vi "_lvcicd_dependencies-Post-Install Custom Action.vi"(10 "Variant":variant) -> (0 "error out":errorcluster)   [LabVIEW 2014]
panel:
  out "data":T1(ring)
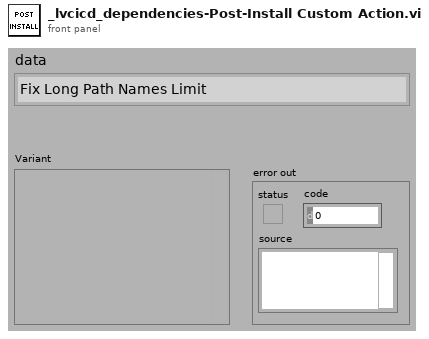
[diagram p1: front panel]
types:
  T1 = enum16{"Fix Long Path Names Limit", "Fix Running Scripts Is Disabled", "-- Exit ---"}
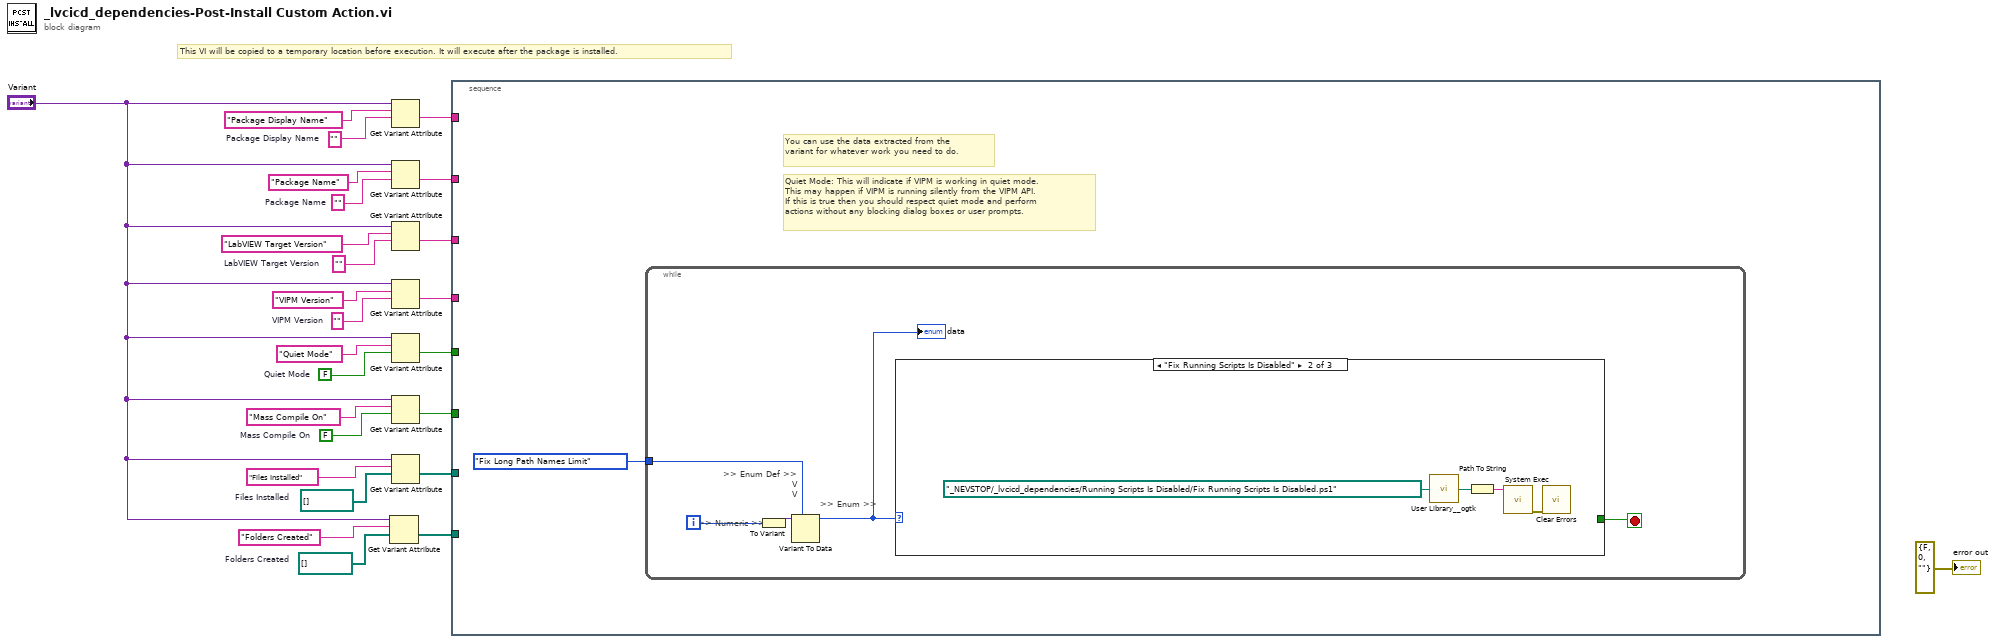
[diagram p0: block diagram]
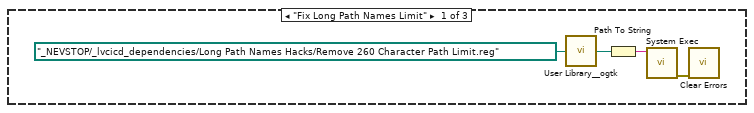
[diagram p2: hidden frame]
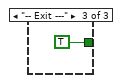
[diagram p3: hidden frame]
diagram:
  w1 = path[] []  # Folders Created
  w2 = path[] []  # Files Installed
  w8 = FALSE  # Mass Compile On
  w9 = ""  # Package Display Name
  w16 = FALSE  # Quiet Mode
  w19 = ""  # VIPM Version
  w21 = ""  # LabVIEW Target Version
  w23 = ""  # Package Name
  # "This VI will be copied to a temporary location before execution. It will execute after the package is installed."
  n1 = Get Variant Attribute(Variant="Variant", name="Folders Created", default value (empty Variant)=w1) -> (value=w6:path[])  [unwired: 1 in, 3 out]
  n2 = Get Variant Attribute(Variant="Variant", name="Package Display Name", default value (empty Variant)=w9) -> (value=w15:string)  [unwired: 1 in, 3 out]
  n3 = Get Variant Attribute(Variant="Variant", name="Package Name", default value (empty Variant)=w23) -> (value=w14:string)  [unwired: 1 in, 3 out]
  n4 = Get Variant Attribute(Variant="Variant", name="LabVIEW Target Version", default value (empty Variant)=w21) -> (value=w13:string)  [unwired: 1 in, 3 out]
  n5 = Get Variant Attribute(Variant="Variant", name="VIPM Version", default value (empty Variant)=w19) -> (value=w12:string)  [unwired: 1 in, 3 out]
  n6 = Get Variant Attribute(Variant="Variant", name="Quiet Mode", default value (empty Variant)=w16) -> (value=w11:bool)  [unwired: 1 in, 3 out]
  n7 = Get Variant Attribute(Variant="Variant", name="Mass Compile On", default value (empty Variant)=w8) -> (value=w10:bool)  [unwired: 1 in, 3 out]
  n8 = Get Variant Attribute(Variant="Variant", name="Files Installed", default value (empty Variant)=w2) -> (value=w5:path[])  [unwired: 1 in, 3 out]
  n9 = stacked-sequence {
    tunnel: w15 -> [_]
    tunnel: w14 -> [_]
    tunnel: w13 -> [_]
    tunnel: w12 -> [_]
    tunnel: w11 -> [_]
    tunnel: w10 -> [_]
    tunnel: w5 -> [_]
    tunnel: w6 -> [_]
    frame #0 {
      # "Quiet Mode: This will indicate if VIPM is working in quiet mode.\nThis may happen if VIPM is running silently from the VIPM API.\nIf this is true then you should respect quiet mode and perform\nactions without any blocking dialog boxes or user prompts."
      # "You can use the data extracted from the variant for whatever work you need to do."
      n10 = while {
        tunnel: T1."Fix Long Path Names Limit" -> [w30]
        i -> [w31]
        stop <- w28 stop-if-true
        # ">> Enum >>"
        # ">> Enum Def >>\n                       V\n                       V"
        # ">> Numeric >>"
        n11 = To Variant(anything=w31) -> (Variant=w32:variant)
        n12 = Variant To Data(type=w30, Variant=w32) -> (data=w29:T1)  [unwired: 1 in, 1 out]
        "data" <- w29
        n13 = case shown="\"Fix Running Scripts Is Disabled\"" w29 {
          tunnel: [_ _ TRUE] -> w28
          frame "Fix Long Path Names Limit" {
            n14 = call <userlib>:"User Library__ogtk.vi"("Relative path (.)"=path "_NEVSTOP/_lvcicd_dependencies/Long Path Names Hacks/Remove 260 Character Path Limit.reg") -> ("User Library (+ Relative)"=w35:path)
            n15 = Path To String(path=w35) -> (string=w34:string)
            n16 = call <vilib>:"System Exec.vi"("command line"=w34) -> ("error out"=w33:errorcluster)  [unwired: 7 in, 3 out]
            n17 = call <vilib>:"Clear Errors.vi"("error in (no error)"=w33) -> ()  [unwired: 5 in, 2 out]
          }
          frame "Fix Running Scripts Is Disabled" {
            n18 = call <userlib>:"User Library__ogtk.vi"("Relative path (.)"=path "_NEVSTOP/_lvcicd_dependencies/Running Scripts Is Disabled/Fix Running Scripts Is Disabled.ps1") -> ("User Library (+ Relative)"=w39:path)
            n19 = Path To String(path=w39) -> (string=w38:string)
            n20 = call <vilib>:"System Exec.vi"("command line"=w38) -> ("error out"=w37:errorcluster)  [unwired: 7 in, 3 out]
            n21 = call <vilib>:"Clear Errors.vi"("error in (no error)"=w37) -> ()  [unwired: 5 in, 2 out]
          }
          frame "-- Exit ---" {
          }
        }
      }
    }
  }
  "error out" <- errorcluster {"status"=FALSE, "code"=0, "source"=""} ("error out")
